vi "Module Timeout--constant.vi"() -> (3 "Module Timeout":i32)   [LabVIEW 2020, in "Paquetes Disponibles.lvlib"]
doc: "A module-wide common value to use as the timeout for various synchronization actions.\n_____\nBased on DQMH Project Template 6.0.0.91."
uses:
  Paquetes Disponibles.lvlib
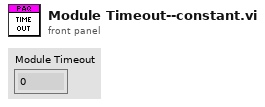
[diagram p1: front panel]
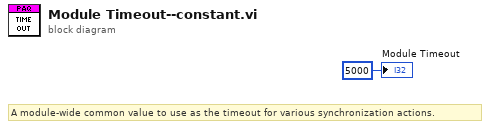
[diagram p0: block diagram]
diagram:
  # "A module-wide common value to use as the timeout for various synchronization actions."
  "Module Timeout" <- 5000 ("Module Timeout")
